vi "Main Host Comms.vi"() -> ()   [LabVIEW 2019]
uses:
  RT Controls/Main Process Commands.ctl
  RT Controls/Main Command Events.ctl
  RT Controls/Main Comm State.ctl
  <vilib>/Utility/error.llb/DialogType.ctl
panel:
  out "main queue":refnum<queue>
  out "state":enum16{"connect", "run", "close"}(ring)
  out "error out":errorcluster
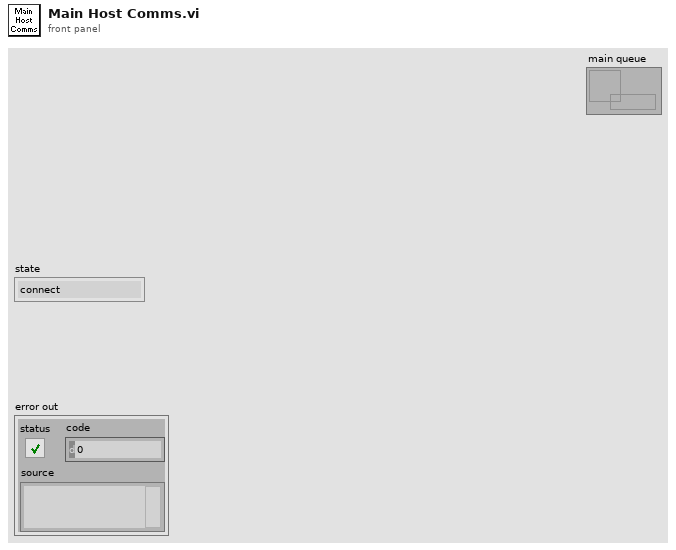
[diagram p1: front panel]
types:
  T1 = typedef "Main Process Commands.ctl" = cluster{"Commands":T2, "Value":variant}
  T2 = typedef "Main Command Events.ctl" = enum16{"Idle", "FullStop", "MainReadConfig", "MainWriteConfig", "OpenUpper", "CloseUpper", "OpenLower", "CloseLower", "SetWatchdogInt", "EnCloudShutDn", "DisCloudShutDn", "SetRainDelay", "EnAutoShutDn", "DisAutoShutDn", "SetRevDelay", "RotToAz", "RotLeft", "RotRight", "RotToHome", "DefineHomePos", "SetHSThres", "SetEncCounts", "SyncClose", "SyncOpen", "SetAZTimLim", "SetAZTol", "AZEncPositive", "AZEncNegative", "RotToCenter"}
  T3 = typedef "Main Comm State.ctl" = enum16{"Init", "Run"}
  T4 = enum16{"Standard", "Buffered", "CRLF", "Immediate"}
  T5 = typedef "DialogType.ctl" = u16
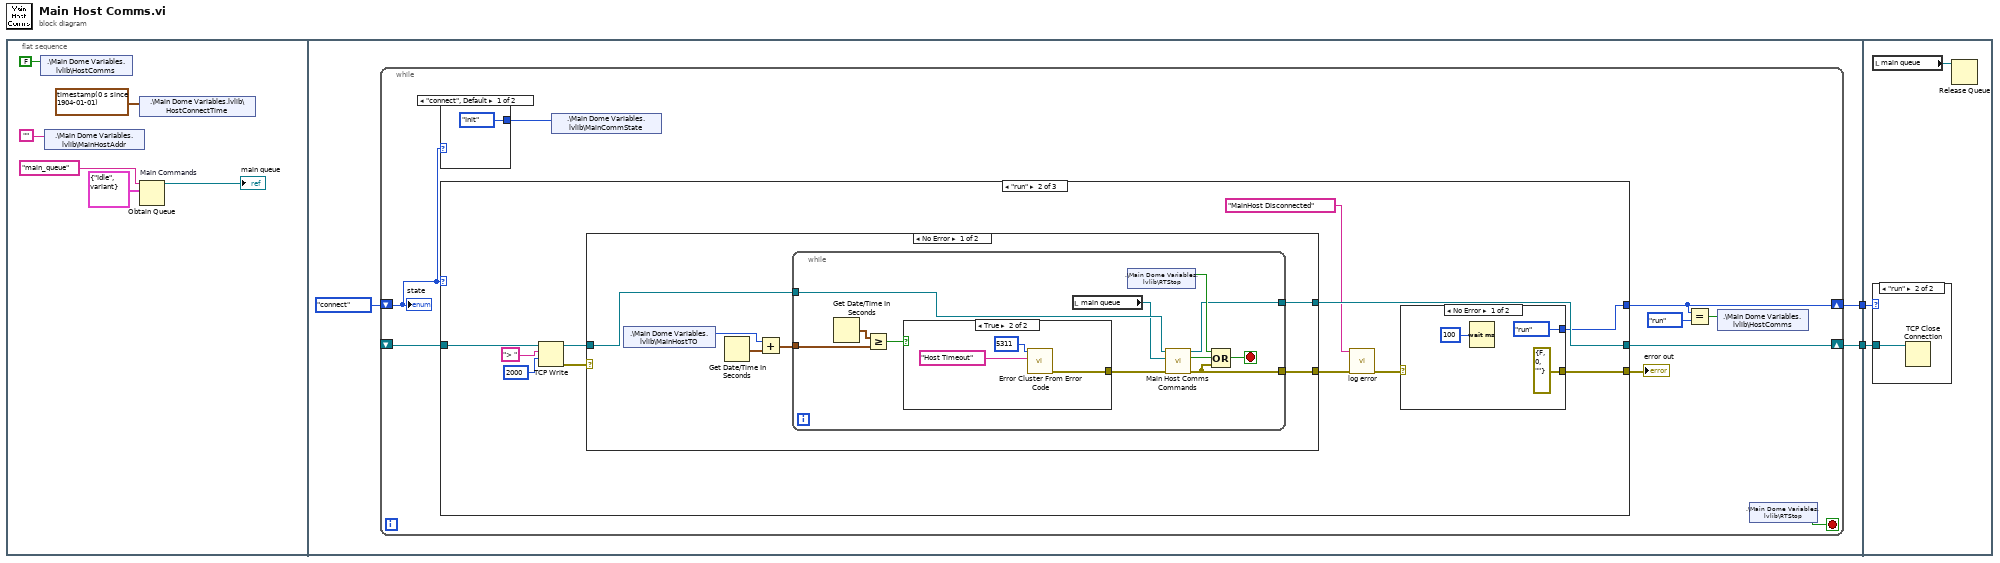
[diagram p0: block diagram]
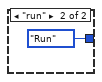
[diagram p2: hidden frame]
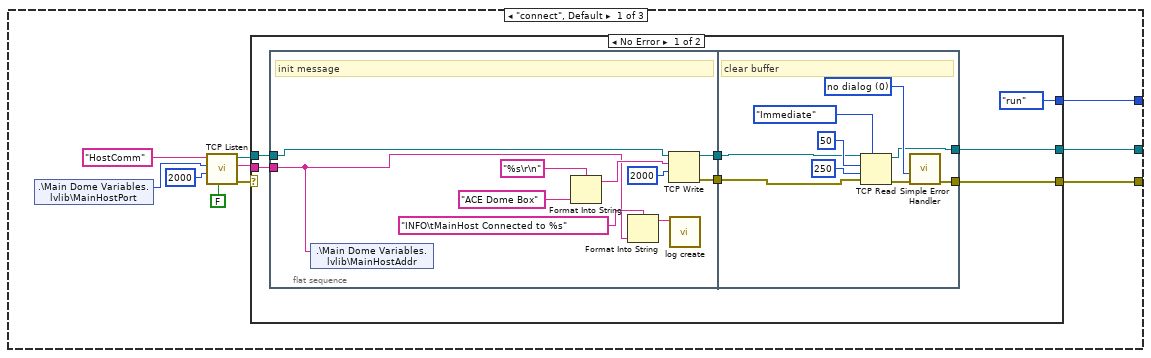
[diagram p3: hidden frame]
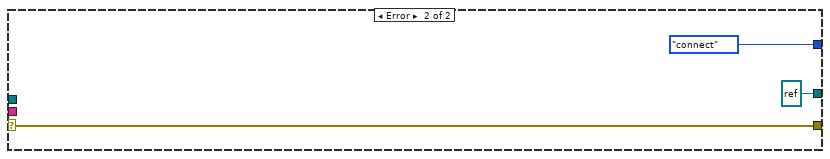
[diagram p4: hidden frame]
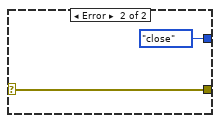
[diagram p5: hidden frame]
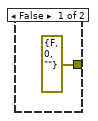
[diagram p6: hidden frame]
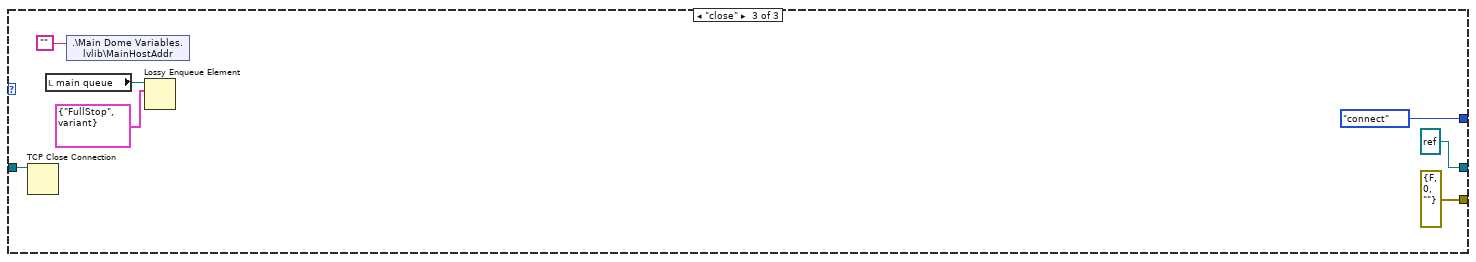
[diagram p8: hidden frame]
diagram:
  n1 = flat-sequence {
    tunnel: [w10] -> w2
    tunnel: [w9] -> w1
    tunnel: w2 -> [w110]
    tunnel: w1 -> [w109]
    frame #0 {
      n2 = shared-variable ".\\Main Dome Variables.lvlib\\HostComms"(FALSE ("HostComms")) -> ()  [unwired: 1 in, 1 out]
      n3 = shared-variable ".\\Main Dome Variables.lvlib\\MainHostAddr"("" ("MainHostAddr")) -> ()  [unwired: 1 in, 1 out]
      n4 = shared-variable ".\\Main Dome Variables.lvlib\\HostConnectTime"(timestamp(0 s since 1904-01-01) ("HostConnectTime")) -> ()  [unwired: 1 in, 1 out]
      n5 = Obtain Queue "Main Commands"(name (unnamed)="main_queue", element data type=T1 {"Commands"=enum."Idle", "Value"=variant} ("ProcessEvents")) -> (queue out=→"main queue":refnum<queue>)  [unwired: 3 in, 2 out]
    }
    frame #1 {
      n6 = while {
        shift-right: [w15] -> w10
        shift-left: enum16{"connect", "run", "close"}."connect" ("y") -> [w13]
        shift-right: [w19] -> w9
        shift-left: _ -> [w18]
        stop <- w20 stop-if-true
        n7 = case shown="\"connect\", Default" w13 {
          tunnel: [Main_Comm_State."Init" ("BoxCommState") Main_Comm_State."Run" ("BoxCommState")] -> w12
          frame "connect", Default {
          }
          frame "run" {
          }
        }
        n8 = case shown="\"run\"" w13 {
          tunnel: [w27 w65 enum16{"connect", "run", "close"}."connect"] -> w15
          tunnel: [w26 w67 refnum<k5> refnum ("connection ID")] -> w19
          tunnel: w18 -> [_ w68 w104]
          tunnel: [w25 w66 errorcluster {"status"=FALSE, "code"=0, "source"=""} ("error IO")] -> w17
          frame "connect", Default {
            n9 = shared-variable ".\\Main Dome Variables.lvlib\\MainHostPort"() -> (w30:u16)  [unwired: 1 in, 1 out]
            n10 = call <vilib>:"TCP Listen.vi"("resolve remote address (T)"=FALSE, "timeout ms (wait forever: -1)"=2000, "port"=w30, "service name"="HostComm") -> ("error out"=w29:errorcluster, "remote address"=w24:string, "connection ID"=w28:refnum<k5>)  [unwired: 1 in, 4 out]
            n11 = case shown="No Error" w29 {
              selector: w29 -> [_ w60]
              tunnel: [enum16{"connect", "run", "close"}."run" enum16{"connect", "run", "close"}."connect"] -> w27
              tunnel: [w35 w60] -> w25
              tunnel: w28 -> [w38 _]
              tunnel: [w34 refnum<k5> refnum ("connection ID")] -> w26
              tunnel: w24 -> [w33 _]
              frame No Error {
                n12 = flat-sequence {
                  tunnel: w38 -> [w46]
                  tunnel: [w45] -> w37
                  tunnel: [w43] -> w36
                  tunnel: w33 -> [w40]
                  tunnel: w37 -> [w51]
                  tunnel: w36 -> [w53]
                  tunnel: [w52] -> w35
                  tunnel: [w50] -> w34
                  frame #0 {
                    # "init message"
                    n13 = shared-variable ".\\Main Dome Variables.lvlib\\MainHostAddr"(w40) -> ()  [unwired: 1 in, 1 out]
                    n14 = Format Into String(format string="%s\r\n", "ACE Dome Box" ("string")) -> (resulting string=w49:string)  [unwired: 2 in, 1 out]
                    n15 = Format Into String(format string="INFO\tMainHost Connected to %s" ("message"), w40) -> (resulting string=w41:string)  [unwired: 2 in, 1 out]
                    n16 = TCP Write(connection ID=w46, data in=w49, 9:2000 ("timeout ms (25000)")) -> (connection ID out=w45:refnum<k5>, error out=w43:errorcluster)  [unwired: 1 in, 1 out]
                    n17 = call "log create.vi"("message"=w41) -> ()  [unwired: 11 in]
                  }
                  frame #1 {
                    w57 = T5 0 items=["no dialog", "OK message", "continue or stop message", "OK message + warnings", "continue/stop + warnings"] ("type of dialog (OK msg:1)")
                    # "clear buffer"
                    n18 = TCP Read(connection ID=w51, bytes to read=50, error in (no error)=w53, 7:T4."Immediate" ("mode (standard)"), 9:250 ("timeout ms (25000)")) -> (connection ID out=w50:refnum<k5>, error out=w58:errorcluster)  [unwired: 1 out]
                    n19 = call <vilib>:"Simple Error Handler.vi"("type of dialog (OK msg:1)"=w57, "error in (no error)"=w58) -> ("error out"=w52:errorcluster)  [unwired: 3 in, 4 out]
                  }
                }
              }
              frame Error {
              }
            }
          }
          frame "run" {
            n20 = TCP Write(connection ID=w68, data in="> " ("string"), 9:2000 ("timeout ms (25000)")) -> (connection ID out=w69:refnum<k5>, error out=w70:errorcluster)  [unwired: 1 in, 1 out]
            n21 = case shown="No Error" w70 {
              selector: w70 -> [_ w100]
              tunnel: w69 -> [w83 w99]
              tunnel: [w82 w99] -> w67
              tunnel: [w81 w100] -> w64
              frame No Error {
                n22 = shared-variable ".\\Main Dome Variables.lvlib\\MainHostTO"() -> (w80:u16)  [unwired: 1 in, 1 out]
                n23 = Get Date/Time In Seconds() -> (seconds since 1Jan1904=w79:timestamp)
                n24 = Add(x=w80, y=w79) -> (x+y=w78:timestamp)
                n25 = while {
                  tunnel: w83 -> [w89]
                  tunnel: w78 -> [w92]
                  tunnel: [w85] -> w82
                  tunnel: [w86] -> w81
                  stop <- w91 stop-if-true
                  n26 = Get Date/Time In Seconds() -> (seconds since 1Jan1904=w94:timestamp)
                  n27 = Greater Or Equal?(x=w94, y=w92) -> (x >= y?=w93:bool)
                  n28 = case shown="True" w93 {
                    tunnel: [errorcluster {"status"=FALSE, "code"=0, "source"=""} ("error out") w96] -> w87
                    frame False {
                    }
                    frame True {
                      n29 = call <vilib>:"Error Cluster From Error Code.vi"("error message (\"\")"="Host Timeout" ("error message (\"\")"), "error code (0)"=5311) -> ("error out"=w96:errorcluster)  [unwired: 7 in]
                    }
                  }
                  n30 = local read "main queue"() -> (w88:refnum<queue>)
                  n31 = shared-variable ".\\Main Dome Variables.lvlib\\RTStop"() -> (w90:bool)  [unwired: 1 in, 1 out]
                  n32 = call "Main Host Comms Commands.vi"("error in"=w87, "main queue"=w88, "tcp in"=w89) -> ("error out"=w86:errorcluster, "processed?"=w84:bool, "tcp out"=w85:refnum<k5>)  [unwired: 6 in]
                  n33 = Compound Arithmetic op=OR(w90, w84, w86) -> (w91:bool)
                }
              }
              frame Error {
              }
            }
            n34 = call "log error.vi"("error in"=w64, "message"="MainHost Disconnected") -> ("error out"=w62:errorcluster)  [unwired: 9 in]
            n35 = case shown="No Error" w62 {
              selector: w62 -> [_ w76]
              tunnel: [enum16{"connect", "run", "close"}."run" enum16{"connect", "run", "close"}."close"] -> w65
              tunnel: [errorcluster {"status"=FALSE, "code"=0, "source"=""} ("error IO") w76] -> w66
              frame No Error {
                n36 = Wait (ms)(milliseconds to wait=u32 100) -> ()  [unwired: 1 out]
              }
              frame Error {
              }
            }
          }
          frame "close" {
            n37 = TCP Close Connection(connection ID=w104) -> ()  [unwired: 2 in, 2 out]
            n38 = local read "main queue"() -> (w102:refnum<queue>)
            n39 = shared-variable ".\\Main Dome Variables.lvlib\\MainHostAddr"("" ("MainHostAddr")) -> ()  [unwired: 1 in, 1 out]
            n40 = Lossy Enqueue Element(queue=w102, element=T1 {"Commands"=enum."FullStop", "Value"=variant} ("event data")) -> ()  [unwired: 1 in, 4 out]
          }
        }
        "error out" <- w17
        n41 = shared-variable ".\\Main Dome Variables.lvlib\\MainCommState"(w12) -> ()  [unwired: 1 in, 1 out]
        n42 = Equal?(x=w15, y=enum16{"connect", "run", "close"}."run") -> (x = y?=w14:bool)
        n43 = shared-variable ".\\Main Dome Variables.lvlib\\HostComms"(w14) -> ()  [unwired: 1 in, 1 out]
        n44 = shared-variable ".\\Main Dome Variables.lvlib\\RTStop"() -> (w20:bool)  [unwired: 1 in, 1 out]
        "state" <- w13
      }
    }
    frame #2 {
      n45 = local read "main queue"() -> (w108:refnum<queue>)
      n46 = case shown="\"run\"" w110 {
        tunnel: w109 -> [_ w111]
        frame "connect", Default {
        }
        frame "run" {
          n47 = TCP Close Connection(connection ID=w111) -> ()  [unwired: 2 in, 2 out]
        }
      }
      n48 = Release Queue(queue=w108) -> ()  [unwired: 2 in, 3 out]
    }
  }
